vi "Write Bit.vi"(8 "error in (no error)":errorcluster, 10 "Bit":bool, 11 "Bit in":refnum<class "Bit.lvclass">) -> (0 "error out":errorcluster, 3 "Bit out":refnum<class "Bit.lvclass">)   [LabVIEW 2016, in "Bit.lvclass"]
uses:
  Bit.lvclass
  Bit.lvclass/Bit.ctl
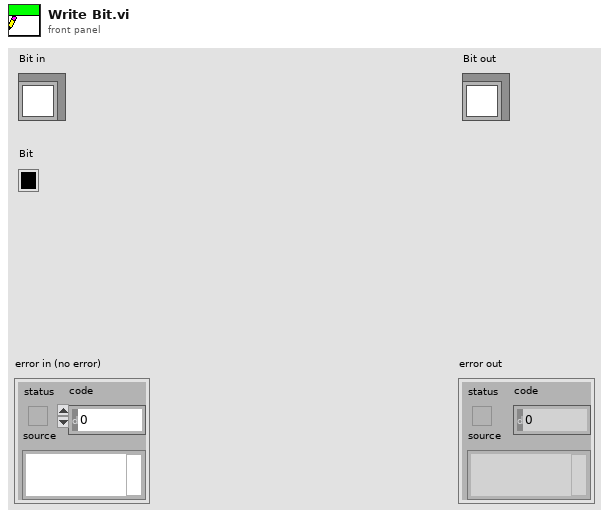
[diagram p1: front panel]
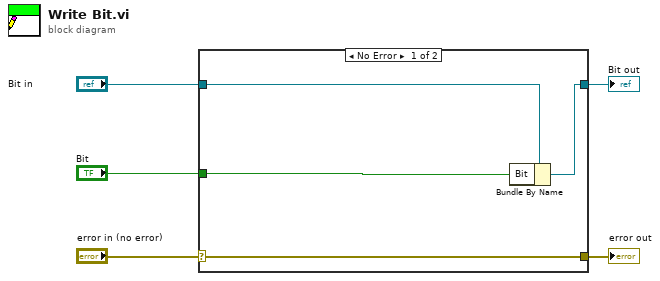
[diagram p0: block diagram]
diagram:
  n1 = case shown="No Error" "error in (no error)" {
    selector: "error in (no error)" -> [w9 w10]
    tunnel: [w9 w10] -> w4
    tunnel: [w7 w11] -> w2
    tunnel: "Bit in" -> [w8 w11]
    tunnel: "Bit" -> [w6 _]
    frame No Error {
      n2 = Bundle By Name(cluster=w8, "Bit"=w6) -> (w7:refnum<class "Bit.lvclass">)
    }
    frame Error {
    }
  }
  "error out" <- w4
  "Bit out" <- w2
